vi "堆芯装卸料图程序.vi"() -> ()   [LabVIEW 2020]
doc: "图片控件可作为用户的绘图界面。本范例主要使用了画笔宽度和样式属性以及子集获取功能。子集获取是指从任意图像中截取一个矩形区域并绘制新图像的功能。"
uses:
  <vilib>/Utility/miscctls.llb/LVRowAndColumnTypeDef.ctl
  <vilib>/Analysis/baseanly.llb/Mean (DBL).vi
  GlobalVariable.vi
  <vilib>/Analysis/NI_AALBase.lvlib
panel:
  in  "操作显示":bool
  out "鼠标列":i32
  out "鼠标指示位置":i32(ring) items=["A"=0, "B"=1, "C"=2, "D"=3, "E"=4, "F"=5, "G"=6, "H"=7, "J"=8, "K"=9, "L"=10, "M"=11, "N"=12, " "=-2, " "=-1]
  in  "操作选项卡":enum32{"装卸料操作", "图操作"}(tab)
  in  "选取数据":bool
  out "波形图":dbl[][](graph)
  in  "当前堆内组件数":i32
  in  "SRC1&SRC2":string[][](array[string])
  in  "Select Pen Attributes":T1={"Width"=1, "Style"=enum."Solid"} caption="手动标记"
  out "Subset":picture caption="局部截图"
  in  "Select Operation":T2(ring) caption="选择操作"
  in  "Pen Color":u32(colorbox)=15671808 caption="标记颜色"
  out "Mouse Position.X":i32
  out "Mouse Position.Y":i32
  out "图层保存":bool
  in  "上一步装料":bool
  in  "下一步装料":bool
  out "PlanTable":string[][](table) caption="汇总表格"
  in  "初始化堆芯图":bool
  in  "保存图与SRC":bool
  out "Draw??":bool caption="绘制？？"
  out "Initial Coordinates":cluster{"Horizontal":i16, "Vertical":i16} caption="初始坐标"
  in  "退出程序":bool caption="停止"
  out "Picture":picture caption="堆芯图"
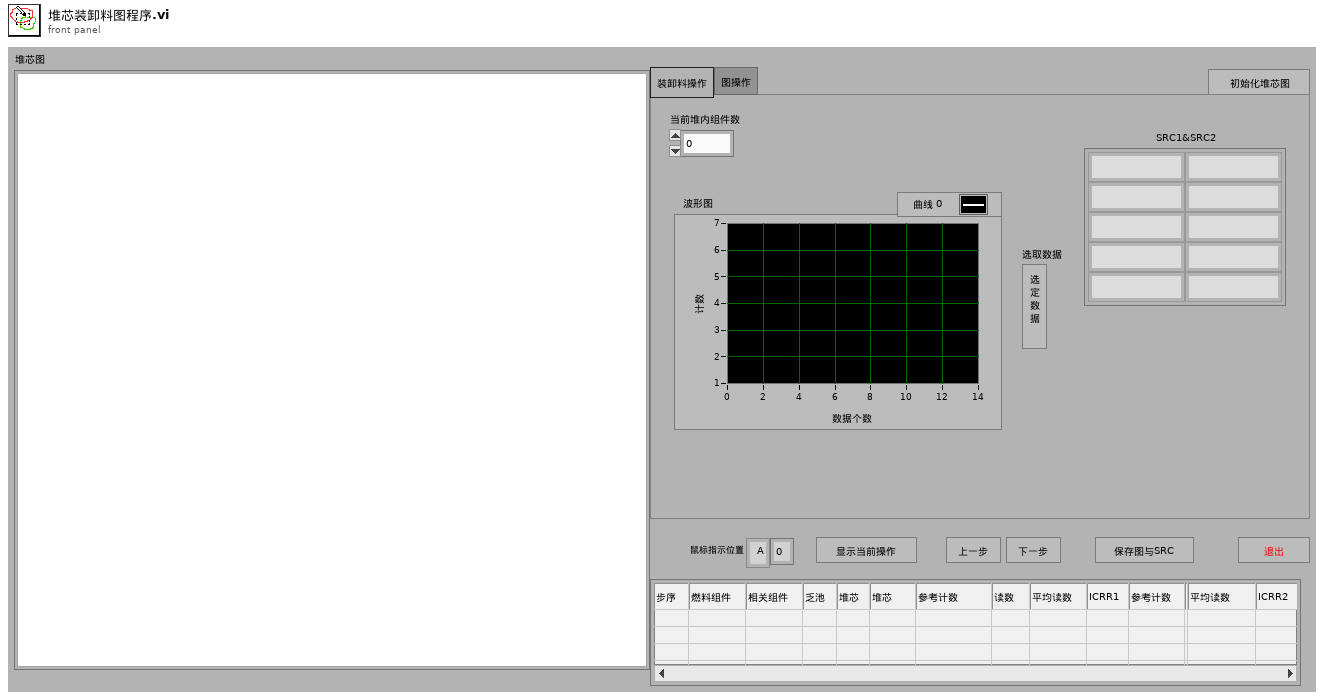
[diagram p1: front panel]
types:
  T1 = cluster{"Width":u16, "Style":enum32{"Solid", "Dash", "Dot", "DashDot", "DashDotDot"}}
  T2 = enum16{"Select Subset", "Draw Line", "Draw Point"}
  T3 = typedef "imagedata.ctl" = cluster{"image type":i32, "image depth":i32, "image":u8[], "mask":u8[], "colors":u32[], "Rectangle":cluster{"left":i16, "top":i16, "right":i16, "bottom":i16}}
  T4 = enum32{"Solid", "Dash", "Dot", "DashDot", "DashDotDot"}
  T5 = typedef "LVMouseTypeDef.ctl" = cluster{"Mouse Position":cluster{"X":i32, "Y":i32}, "Mouse Modifiers":cluster{"Button Down":bool, "Shift Mod":bool, "Menu Mod":bool, "Option Mod":bool}}
  T6 = typedef "LVRowAndColumnTypeDef.ctl" = cluster{"Row":i32, "Column":i32}
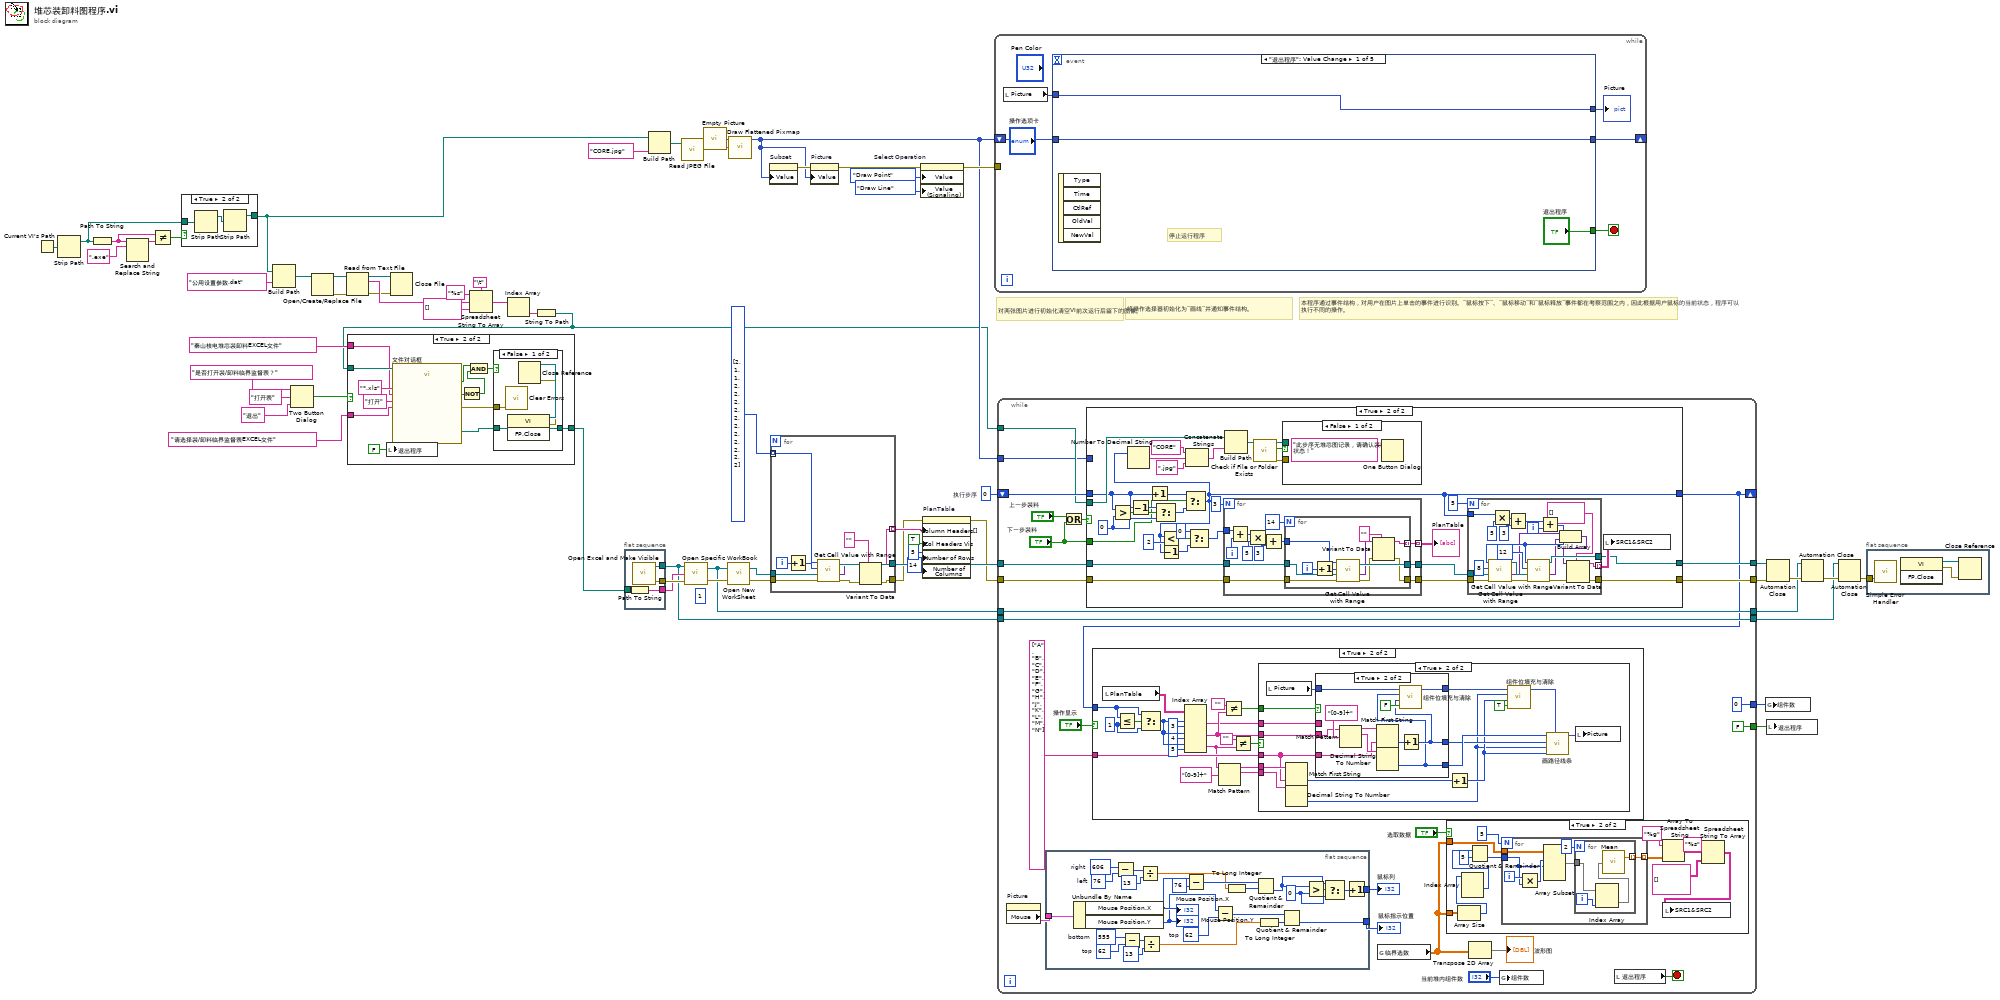
[diagram p0: block diagram]
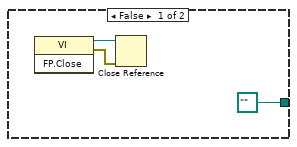
[diagram p2: hidden frame]
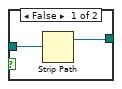
[diagram p4: hidden frame]
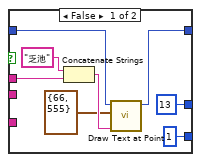
[diagram p8: hidden frame]
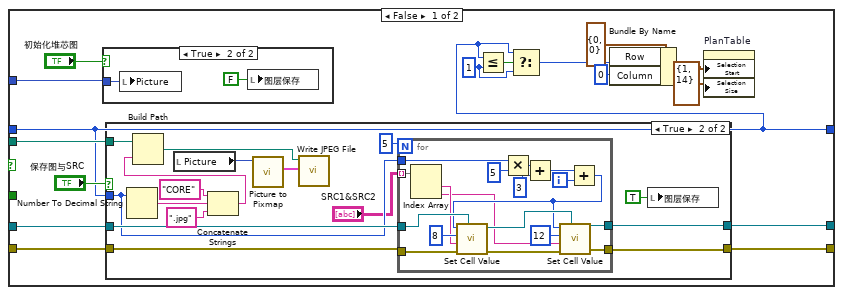
[diagram p9: hidden frame]
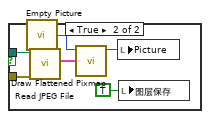
[diagram p12: hidden frame]
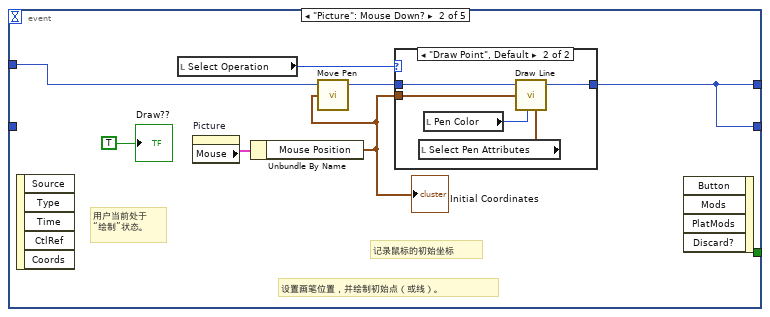
[diagram p13: hidden frame]
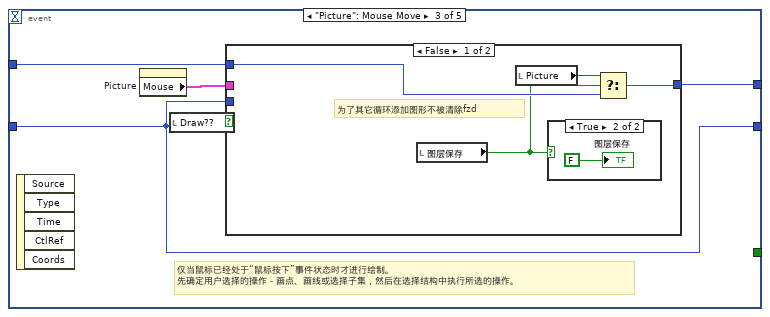
[diagram p15: hidden frame]
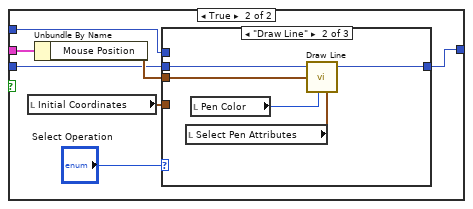
[diagram p17: hidden frame]
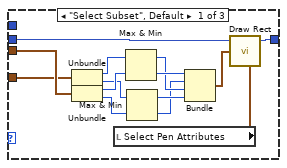
[diagram p18: hidden frame]
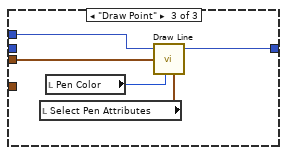
[diagram p19: hidden frame]
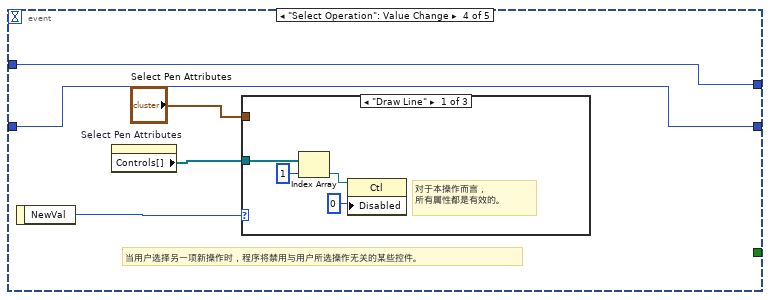
[diagram p20: hidden frame]
diagram:
  w32 = 0  # 执行步序
  (unwired) 1 ("Sheet")
  # "本程序通过事件结构，对用户在图片上单击的事件进行识别。“鼠标按下”、“鼠标移动”和“鼠标释放”事件都在考察范围之内，因此根据用户鼠标的当前状态，程序可以执行不同的操作。"
  # "将操作选择器初始化为“画线”并通知事件结构。"
  # "对两张图片进行初始化清空VI前次运行后留下的图像。"
  n1 = Current VI's Path() -> (path=w27:path)
  n2 = Strip Path(path=w27) -> (stripped path=w22:path)  [unwired: 1 out]
  n3 = Path To String(path=w22) -> (string=w24:string)
  n4 = Search and Replace String(input string=w24, search string=".exe" ("搜索字符串")) -> (result string=w25:string)  [unwired: 6 in, 3 out]
  n5 = Not Equal?(x=w24, y=w25) -> (x != y?=w23:bool)
  n6 = case shown="True" w23 {
    tunnel: w22 -> [w64 w67]
    tunnel: [w63 w65] -> w3
    frame False {
      n7 = Strip Path(path=w64) -> (stripped path=w63:path)  [unwired: 1 out]
    }
    frame True {
      n8 = Strip Path(path=w67) -> (stripped path=w66:path)  [unwired: 1 out]
      n9 = Strip Path(path=w66) -> (stripped path=w65:path)  [unwired: 1 out]
    }
  }
  n10 = Build Path(base path=w3, name or relative path="公用设置参数.dat") -> (appended path=w9:path)
  n11 = Two Button Dialog(message="是否打开装/卸料临界监督表？", 1:"退出" ("message"), 2:"打开表" ("message")) -> (T button?=w19:bool)
  n12 = Open/Create/Replace File(file path (use dialog)=w9) -> (refnum out=w12:refnum<file>, error out=w13:errorcluster)  [unwired: 5 in, 1 out]
  n13 = Read from Text File(file (use dialog)=w12, error in=w13) -> (refnum out=w11:refnum<file>, text=w17:string, error out=w10:errorcluster)  [unwired: 1 in, 2 out]
  n14 = Close File(refnum=w11, error in=w10) -> ()  [unwired: 2 out]
  n15 = Spreadsheet String To Array(delimiter (Tab)="\t", format string="%s", spreadsheet string=w17, array type (2D Dbl)=string[] [] ("添加的数组")) -> (array=w18:string[])
  n16 = Index Array(array=w18) -> (element=w7:string)  [unwired: 1 in]
  n17 = String To Path(string=w7) -> (path=w2:path)
  n18 = case shown="True" w19 {
    tunnel: w2 -> [_ w83]
    tunnel: "请选择装/卸料临界监督表EXCEL文件" ("prompt") -> [_ w79]
    tunnel: "秦山核电堆芯装卸料EXCEL文件" ("pattern label") -> [_ w78]
    tunnel: [path "" ("selected path") w76] -> w1
    frame False {
      n19 = invoke class="VI" method="FP.Close"() -> (reference out=w69:refnum<vi>, error out=w68:errorcluster)  [unwired: 3 in, 1 out]
      n20 = Close Reference(reference=w69, error in (no error)=w68) -> ()  [unwired: 1 out]
    }
    frame True {
      n21 = local write "退出程序"(FALSE ("退出程序")) -> ()
      n22 = call "文件对话框"("start path"=w83, "prompt"=w79, "button label"="打开", "pattern (all files)"="*.xls", "pattern label"=w78) -> ("selected path"=w77:path, "exists"=w74:bool, "cancelled"=w75:bool, "error out"=w71:errorcluster)  [unwired: 7 in]
      n23 = Not(x=w75) -> (.not. x?=w73:bool)
      n24 = And(x=w74, y=w73) -> (x .and. y?=w72:bool)
      n25 = case shown="False" w72 {
        tunnel: w77 -> [w87 w88]
        tunnel: [w87 w88] -> w76
        tunnel: w71 -> [w86 _]
        frame False {
          n26 = call <vilib>:"Clear Errors.vi"("error in (no error)"=w86) -> ()  [unwired: 5 in, 2 out]
          n27 = invoke class="VI" method="FP.Close"() -> (reference out=w85:refnum<vi>, error out=w84:errorcluster)  [unwired: 3 in, 1 out]
          n28 = Close Reference(reference=w85, error in (no error)=w84) -> ()  [unwired: 1 out]
        }
        frame True {
        }
      }
    }
  }
  n29 = flat-sequence {
    tunnel: [w92] -> w53
    tunnel: [w91] -> w52
    tunnel: [w90] -> w46
    tunnel: w1 -> [w89]
    frame #0 {
      n30 = Path To String(path=w89) -> (string=w91:string)
      n31 = call "Open Excel and Make Visible.vi"() -> ("error out"=w92:errorcluster, "Excel._Application"=w90:refnum<k7>)  [unwired: 2 in]
    }
  }
  n32 = Build Path(base path=w3, name or relative path="CORE.jpg" ("名称或相对路径")) -> (appended path=w57:path)
  n33 = call <vilib>:"Read JPEG File.vi"("path to JPEG file"=w57) -> ("image data"=w55:T3)  [unwired: 8 in, 2 out]
  n34 = call "Open Specific WorkBook.vi"("error in (no error)"=w53, "Filename of Workbook"=w52, "Excel._Application"=w46) -> ("error out"=w43:errorcluster, "Excel._Workbook"=w42:refnum<k7>)
  n35 = call "Empty Picture"() -> ("empty picture"=w54:picture)
  n36 = call "Open New WorkSheet.vi"("error in (no error)"=w43, "Excel._Workbook"=w42) -> ("error out"=w40:errorcluster, "Excel._Worksheet"=w38:refnum<k7>)  [unwired: 1 in]
  n37 = call <vilib>:"Draw Flattened Pixmap.vi"("image data"=w55, "picture"=w54) -> ("new picture"=w41:picture)  [unwired: 7 in]
  n38 = property on="Subset" class="Pict"("Value"=w41) -> (error out=w58:errorcluster)  [unwired: 2 in, 1 out]
  n39 = for {
    tunnel: w40 -> [w103]
    tunnel: [w95] -> w34
    tunnel: [w102] -> w39
    tunnel: w38 -> [w101]
    tunnel: i32[] [2, 1, 1, 2, 2, 2, 2, 2, 2, 2, 2, 2, 2, 2] -> [w98] mode=indexing
    tunnel: [w93] -> w35 mode=indexing
    i -> [w100]
    n40 = Increment(x=w100) -> (x+1=w99:i32)
    n41 = call "Get Cell Value with Range.vi"("error in (no error)"=w103, "Excel._Worksheet"=w101, "Col"=w99, "Row"=w98) -> ("error out"=w96:errorcluster, "Data Out"=w97:variant, "Excel._Worksheet"=w102:refnum<k7>)  [unwired: 1 out]
    n42 = Variant To Data(error in=w96, type="" ("Workbook Name"), Variant=w97) -> (data=w93:string, error out=w95:errorcluster)
  }
  n43 = property on="Picture" class="Pict"(error in=w58, "Value"=w41) -> (error out=w59:errorcluster)  [unwired: 1 in, 1 out]
  n44 = property on="Select Operation" class="Enum (strict)"(error in=w59, "Value"=T2."Draw Point" ("Select Your Operation"), "Value (Signaling)"=T2."Draw Line" ("Select Your Operation")) -> (error out=w62:errorcluster)  [unwired: 1 in, 1 out]
  n45 = property on="PlanTable" class="Tbl (strict)"(error in=w34, "Column Headers[]"=w35, "Col Headers Vis"=TRUE ("显示项:显示列首"), "Number of Rows"=u32 5 ("行数"), "Number of Columns"=u32 14 ("列数")) -> (error out=w33:errorcluster)  [unwired: 1 in, 1 out]
  n46 = while {
    shift-right: [w105] -> _
    shift-left: w41 -> [w104]
    tunnel: w62 -> [_]
    stop <- w108 stop-if-true
    n47 = local read "Picture"() -> (w107:picture)
    n48 = event shown="[0] \"退出程序\": Value Change" {
      selector: _ -> [_ _ _ _ _]
      dyn-events: _ -> [_ _ _ _ _]
      timeout: _ -> [_ _ _ _ _]
      tunnel: ["退出程序" _ _ _ _] -> w108
      tunnel: [w110 w114 w127 w169 w189] -> w106
      tunnel: w107 -> [w110 w116 w126 w169 w191]
      tunnel: [w109 w114 w125 w166 w189] -> w105
      tunnel: w104 -> [w109 _ w125 w166 w190]
      event "退出程序": Value Change {
        # "停止运行程序"
        n49 = event-data() -> ()  [unwired: 1 in, 5 out]
      }
      event "Picture": Mouse Down? {
        # "设置画笔位置，并绘制初始点（或线）。"
        # "记录鼠标的初始坐标"
        # "用户当前处于\n“绘制”状态。"
        n50 = event-data() -> ()  [unwired: 1 in, 5 out]
        n51 = local read "Select Operation"() -> (w112:T2)
        n52 = property on="Picture" class="Pict"() -> ("Mouse"=w118:T5)  [unwired: 2 in, 2 out]
        n53 = Unbundle By Name(w118) -> ("Mouse Position"=w113:cluster{"X":i32, "Y":i32})
        "Initial Coordinates" <- w113
        n54 = call <vilib>:"Move Pen.vi"("new position"=w113, "picture"=w116) -> ("new picture"=w115:picture)  [unwired: 3 in]
        n55 = case shown="\"Draw Point\", Default" w112 {
          tunnel: w115 -> [w119 w124]
          tunnel: [w119 w123] -> w114
          tunnel: w113 -> [_ w122]
          frame "Select Subset" {
          }
          frame "Draw Point", Default {
            n56 = local read "Select Pen Attributes"() -> (w121:T1)
            n57 = local read "Pen Color"() -> (w120:u32)
            n58 = call <vilib>:"Draw Line.vi"("picture"=w124, "end point"=w122, "color(black)"=w120, "pen"=w121) -> ("new picture"=w123:picture)  [unwired: 5 in]
          }
        }
        n59 = event-data() -> ()  [unwired: 5 in, 1 out]
        "Draw??" <- TRUE ("Draw??")
      }
      event "Picture": Mouse Move {
        # "仅当鼠标已经处于“鼠标按下”事件状态时才进行绘制。\n先确定用户选择的操作－画点、画线或选择子集，然后在选择结构中执行所选的操作。"
        n60 = event-data() -> ()  [unwired: 1 in, 5 out]
        n61 = property on="Picture" class="Pict"() -> ("Mouse"=w128:T5)  [unwired: 2 in, 2 out]
        n62 = local read "Draw??"() -> (w129:bool)
        n63 = case shown="False" w129 {
          tunnel: w126 -> [w132 w140]
          tunnel: w128 -> [_ w139]
          tunnel: [w133 w136] -> w127
          tunnel: w125 -> [_ w135]
          frame False {
            # "为了其它循环添加图形不被清除fzd"
            n64 = local read "图层保存"() -> (w130:bool)
            n65 = local read "Picture"() -> (w131:picture)
            n66 = case shown="True" w130 {
              frame False {
              }
              frame True {
                "图层保存" <- FALSE ("图层保存")
              }
            }
            n67 = Select(t=w131, s=w130, f=w132) -> (s? t:f=w133:picture)
          }
          frame True {
            n68 = local read "Initial Coordinates"() -> (w138:cluster{"Horizontal":i16, "Vertical":i16})
            n69 = Unbundle By Name(w139) -> ("Mouse Position"=w137:cluster{"X":i32, "Y":i32})
            n70 = case shown="\"Draw Line\"" "Select Operation" {
              tunnel: w140 -> [_ _ w162]
              tunnel: w138 -> [w154 _ _]
              tunnel: w137 -> [w155 w159 w163]
              tunnel: [w152 w160 w165] -> w136
              tunnel: w135 -> [w151 w157 _]
              frame "Select Subset", Default {
                n71 = Unbundle(w154) -> ("Horizontal"=w149:i16, "Vertical"=w145:i16)
                n72 = Unbundle(w155) -> ("X"=w148:i32, "Y"=w144:i32)
                n73 = local read "Select Pen Attributes"() -> (w150:T1)
                n74 = Max & Min(x=w149, y=w148) -> (max(x,y)=w146:i32, min(x,y)=w147:i32)
                n75 = Max & Min(x=w145, y=w144) -> (max(x,y)=w143:i32, min(x,y)=w142:i32)
                n76 = Bundle(w147, w142, w146, w143) -> (w153:cluster{i32, i32, i32, i32})  [unwired: 1 in]
                n77 = call <vilib>:"Draw Rect.vi"("picture"=w151, "rect"=w153, "pen"=w150) -> ("new picture"=w152:picture)  [unwired: 6 in]
              }
              frame "Draw Line" {
                n78 = local read "Select Pen Attributes"() -> (w158:T1)
                n79 = local read "Pen Color"() -> (w156:u32)
                n80 = call <vilib>:"Draw Line.vi"("picture"=w157, "end point"=w159, "color(black)"=w156, "pen"=w158) -> ("new picture"=w160:picture)  [unwired: 5 in]
              }
              frame "Draw Point" {
                n81 = local read "Select Pen Attributes"() -> (w164:T1)
                n82 = local read "Pen Color"() -> (w161:u32)
                n83 = call <vilib>:"Draw Line.vi"("picture"=w162, "end point"=w163, "color(black)"=w161, "pen"=w164) -> ("new picture"=w165:picture)  [unwired: 5 in]
              }
            }
          }
        }
      }
      event "Select Operation": Value Change {
        # "当用户选择另一项新操作时，程序将禁用与用户所选操作无关的某些控件。"
        n84 = event-data() -> ("NewVal"=w170:T2)  [unwired: 1 in]
        n85 = property on="Select Pen Attributes" class="Clust (strict)"() -> ("Controls[]"=w168:refnum<vi>[])  [unwired: 2 in, 2 out]
        n86 = case shown="\"Draw Line\"" w170 {
          tunnel: w168 -> [w174 w181 w188]
          tunnel: "Select Pen Attributes" -> [_ w176 w183]
          frame "Draw Line" {
            # "对于本操作而言，\n所有属性都是有效的。"
            n87 = Index Array(array=w174, index=1) -> (element=w172:refnum<vi>)
            n88 = property class="Ctl"(reference=w172, "Disabled"=u8 0) -> ()  [unwired: 1 in, 2 out]
          }
          frame "Draw Point" {
            # "样式属性与本操作无关。\n因此可以禁用该控件\n并将其值锁定于Solid。"
            n89 = Index Array(array=w181, index=1) -> (element=w179:refnum<vi>)
            n90 = Bundle By Name(cluster=w176, "Style"=T4."Solid") -> (w175:T1)
            n91 = property class="Ctl"(reference=w179, "Disabled"=u8 2) -> ()  [unwired: 1 in, 2 out]
            n92 = property on="Select Pen Attributes" class="Clust (strict)"("Value"=w175) -> ()  [unwired: 2 in, 2 out]
          }
          frame "Select Subset" {
            # "用户选择子集时，程序将选框样式锁定于Dash。"
            n93 = Index Array(array=w188, index=1) -> (element=w186:refnum<vi>)
            n94 = Bundle By Name(cluster=w183, "Style"=T4."Dash") -> (w182:T1)
            n95 = property class="Ctl"(reference=w186, "Disabled"=u8 2) -> ()  [unwired: 1 in, 2 out]
            n96 = property on="Select Pen Attributes" class="Clust (strict)"("Value"=w182) -> ()  [unwired: 2 in, 2 out]
          }
        }
      }
      event "Picture": Mouse Up {
        # "用户绘制完毕后，程序完成该项操作。只需要完成该项操作，\n“选择子集”操作就全部完成了。"
        # "绘制完成"
        n97 = event-data() -> ()  [unwired: 1 in, 1 out]
        n98 = local read "Select Operation"() -> (w193:T2)
        n99 = local write "Draw??"(FALSE ("Draw??")) -> ()
        n100 = case shown="\"Draw Point\"" w193 {
          tunnel: w191 -> [_ w210 w211]
          tunnel: [w194 w210 w211] -> w189
          tunnel: w190 -> [w194 _ _]
          frame "Select Subset", Default {
            # "获取选框的坐标，然后从主图片中抽取子集，并在子集显示控件中\n将该子集绘制为一张新图片。"
            n101 = local read "Initial Coordinates"() -> (w207:cluster{"Horizontal":i16, "Vertical":i16})
            n102 = property on="Picture" class="Pict"() -> ("Mouse"=w208:T5)  [unwired: 2 in, 2 out]
            n103 = Unbundle By Name(w208) -> ("Mouse Position.X"=w197:i32, "Mouse Position.Y"=w195:i32)
            n104 = Unbundle By Name(w207) -> ("Horizontal"=w198:i16, "Vertical"=w196:i16)
            n105 = Max & Min(x=w198, y=w197) -> (max(x,y)=w202:i32, min(x,y)=w201:i32)
            n106 = Max & Min(x=w196, y=w195) -> (max(x,y)=w200:i32, min(x,y)=w199:i32)
            n107 = call <vilib>:"Picture to Pixmap.vi"("picture"=w194) -> ("image data"=w209:T3)  [unwired: 9 in, 1 out]
            n108 = Bundle(w201, w199, w202, w200) -> (w206:cluster{i32, i32, i32, i32})  [unwired: 1 in]
            n109 = call <vilib>:"Get Image Subset.vi"("subset rect"=w206, "image data"=w209) -> ("image subset"=w205:T3)  [unwired: 4 in, 1 out]
            n110 = call "Empty Picture"() -> ("empty picture"=w203:picture)
            n111 = call <vilib>:"Draw Flattened Pixmap.vi"("image data"=w205, "picture"=w203) -> ("new picture"=→"Subset":picture)  [unwired: 7 in]
          }
          frame "Draw Line" {
          }
          frame "Draw Point" {
          }
        }
      }
    }
    "Picture" <- w106
  }
  n112 = while {
    tunnel: [w236] -> w48
    tunnel: [w235] -> w45
    tunnel: [w234] -> w47
    tunnel: w39 -> [w233]
    tunnel: w46 -> [w234]
    tunnel: [w231] -> w44
    tunnel: w33 -> [w232]
    tunnel: w42 -> [w231]
    tunnel: w41 -> [w224]
    shift-right: [w214] -> _
    shift-left: w32 -> [w226]
    tunnel: w2 -> [w225]
    tunnel: [0 ("组件数")] -> w31
    tunnel: [FALSE ("退出程序")] -> w30
    stop <- w220 stop-if-true
    n113 = property on="Picture" class="Pict"() -> ("Mouse"=w230:T5)  [unwired: 2 in, 2 out]
    n114 = flat-sequence {
      tunnel: w230 -> [w285]
      tunnel: [w266] -> w218
      tunnel: [w261] -> w217
      frame #0 {
        w263 = 0 ("y")
        w271 = i16 555  # bottom
        w268 = i16 62  # top
        w272 = i16 62  # top
        w275 = i16 606  # right
        w274 = i16 76  # left
        n115 = Unbundle By Name(w285) -> ("Mouse Position.X"=w284:i32, "Mouse Position.Y"=w283:i32)
        "Mouse Position.X" <- w284
        "Mouse Position.Y" <- w283
        n116 = Subtract(x=w275, y=w274) -> (x-y=w276:i16)
        n117 = Subtract(x=w271, y=w268) -> (x-y=w269:i16)
        n118 = Divide(x=w276, y=i16 13) -> (x/y=w273:dbl)
        n119 = Divide(x=w269, y=i16 13) -> (x/y=w267:dbl)
        n120 = Subtract(x=w284, y=76) -> (x-y=w282:i32)
        n121 = Subtract(x=w283, y=w272) -> (x-y=w281:i32)
        n122 = To Long Integer(number=w273) -> (32bit integer=w279:i32)
        n123 = Quotient & Remainder(x=w282, y=w279) -> (floor(x/y)=w264:i32)  [unwired: 1 out]
        n124 = To Long Integer(number=w267) -> (32bit integer=w280:i32)
        n125 = Quotient & Remainder(x=w281, y=w280) -> (floor(x/y)=w266:i32)  [unwired: 1 out]
        n126 = Greater?(x=w264, y=w263) -> (0:w265:bool)
        n127 = Select(t=w264, s=w265, f=w263) -> (s? t:f=w262:i32)
        n128 = Increment(x=w262) -> (x+1=w261:i32)
      }
    }
    n129 = Or(x="上一步装料", y="下一步装料") -> (x .or. y?=w228:bool)
    n130 = case shown="True" w228 {
      tunnel: [w351 w415] -> w236
      tunnel: [w350 w406] -> w235
      tunnel: w233 -> [w353 w425]
      tunnel: w232 -> [w352 w424]
      tunnel: w226 -> [w341 w396]
      tunnel: [w341 w394] -> w214
      tunnel: "下一步装料" -> [_ w408]
      tunnel: w225 -> [w354 w401]
      tunnel: w224 -> [w348 _]
      frame False {
        w343 = 1 ("y")
        n131 = case shown="True" "初始化堆芯图" {
          tunnel: w348 -> [_ w357]
          frame False {
          }
          frame True {
            n132 = local write "Picture"(w357) -> ()
            n133 = local write "图层保存"(FALSE ("图层保存")) -> ()
          }
        }
        n134 = case shown="True" "保存图与SRC" {
          tunnel: w341 -> [_ w362]
          tunnel: w354 -> [_ w373]
          tunnel: w353 -> [w358 w367]
          tunnel: w352 -> [w359 w365]
          tunnel: [w359 w366] -> w351
          tunnel: [w358 w363] -> w350
          frame False {
          }
          frame True {
            n135 = Number To Decimal String(number=w362) -> (decimal integer string=w371:string)  [unwired: 1 in]
            n136 = local read "Picture"() -> (w374:picture)
            n137 = Concatenate Strings("CORE" ("字符串"), w371, ".jpg" ("字符串")) -> (w369:string)
            n138 = Build Path(base path=w373, name or relative path=w369) -> (appended path=w368:path)
            n139 = call <vilib>:"Picture to Pixmap.vi"("picture"=w374) -> ("image data"=w375:T3)  [unwired: 9 in, 1 out]
            n140 = call <vilib>:"Write JPEG File.vi"("image data"=w375, "path to JPEG file"=w368) -> ()  [unwired: 8 in, 2 out]
            n141 = for {
              N: 5 -> [_]
              tunnel: w365 -> [w393]
              tunnel: w367 -> [w392]
              tunnel: [w381] -> w366
              tunnel: [w389] -> w363
              tunnel: w362 -> [w380]
              tunnel: "SRC1&SRC2" -> [w379] mode=indexing
              i -> [w382]
              n142 = Index Array(array=w379) -> (element #1=w377:string, element #2=w376:string)  [unwired: 2 in]
              n143 = Multiply(x=w380, y=5) -> (x*y=w385:i32)
              n144 = Add(x=w385, y=3) -> (x+y=w383:i32)
              n145 = Add(x=w383, y=w382) -> (x+y=w378:i32)
              n146 = call "Set Cell Value.vi"("Excel._Worksheet"=w392, "error in (no error)"=w393, 6:w377, "Col"=8, "Row"=w378) -> ("error out"=w391:errorcluster, "Excel._Worksheet"=w390:refnum<k7>)  [unwired: 1 in, 1 out]
              n147 = call "Set Cell Value.vi"("Excel._Worksheet"=w390, "error in (no error)"=w391, 6:w376, "Col"=12, "Row"=w378) -> ("error out"=w381:errorcluster, "Excel._Worksheet"=w389:refnum<k7>)  [unwired: 1 in, 1 out]
            }
            n148 = local write "图层保存"(TRUE ("图层保存")) -> ()
          }
        }
        n149 = Less Or Equal?(x=w341, y=w343) -> (x <= y?=w342:bool)
        n150 = Select(t=w341, s=w342, f=w343) -> (s? t:f=w340:i32)
        n151 = Bundle By Name(cluster=T6 {"Row"=0, "Column"=0} ("选择区域起始"), "Row"=w340, "Column"=0) -> (w345:T6)
        n152 = property on="PlanTable" class="Tbl (strict)"("Selection Start"=w345, "Selection Size"=T6 {"Row"=1, "Column"=14} ("选择区域大小")) -> ()  [unwired: 2 in, 2 out]
      }
      frame True {
        w420 = 0 ("y")
        n153 = Greater?(x=w396, y=w420) -> (0:w422:bool)
        n154 = Decrement(x=w396) -> (x-1=w421:i32)
        n155 = Increment(x=w396) -> (x+1=w423:i32)
        n156 = Select(t=w421, s=w422, f=w420) -> (s? t:f=w419:i32)
        n157 = Select(t=w423, s=w408, f=w419) -> (s? t:f=w394:i32)
        n158 = Number To Decimal String(number=w394) -> (decimal integer string=w403:string)  [unwired: 1 in]
        n159 = Less?(x=w394, y=2) -> (x < y?=w412:bool)
        n160 = Decrement(x=w394) -> (x-1=w409:i32)
        n161 = Concatenate Strings("CORE" ("字符串"), w403, ".jpg" ("字符串")) -> (w405:string)
        n162 = Select(t=0 ("y"), s=w412, f=w409) -> (s? t:f=w410:i32)
        n163 = for {
          N: 3 -> [_]
          tunnel: [w466] -> w417
          tunnel: [w465] -> w416
          tunnel: w425 -> [w464]
          tunnel: w424 -> [w463]
          tunnel: [w461] -> w395 mode=indexing
          tunnel: w410 -> [w454]
          i -> [w460]
          n164 = Add(x=w454, y=w460) -> (x+y=w455:i32)
          n165 = Multiply(x=w455, y=5) -> (x*y=w458:i32)
          n166 = Add(x=w458, y=3) -> (x+y=w456:i32)
          n167 = for {
            N: 14 -> [_]
            tunnel: [w468] -> w466
            tunnel: [w477] -> w465
            tunnel: w464 -> [w476]
            tunnel: w463 -> [w475]
            tunnel: w456 -> [w472]
            tunnel: [w467] -> w461 mode=indexing
            i -> [w473]
            n168 = Increment(x=w473) -> (x+1=w474:i32)
            n169 = call "Get Cell Value with Range.vi"("error in (no error)"=w475, "Excel._Worksheet"=w476, "Col"=w474, "Row"=w472) -> ("error out"=w469:errorcluster, "Data Out"=w470:variant, "Excel._Worksheet"=w477:refnum<k7>)  [unwired: 1 out]
            n170 = Variant To Data(error in=w469, type="" ("Workbook Name"), Variant=w470) -> (data=w467:string, error out=w468:errorcluster)
          }
        }
        "PlanTable" <- w395
        n171 = Build Path(base path=w401, name or relative path=w405) -> (appended path=w400:path)
        n172 = call <vilib>:"Check if File or Folder Exists.vi"("path"=w400) -> ("error out"=w398:errorcluster, "file or folder exists?"=w397:bool, "dup path"=w399:path)  [unwired: 8 in]
        n173 = case shown="False" w397 {
          tunnel: w399 -> [_ w430]
          tunnel: w398 -> [_ w429]
          frame False {
            n174 = One Button Dialog(message="此步序无堆芯图记录，请确认装料状态！" ("消息")) -> ()  [unwired: 1 in, 1 out]
          }
          frame True {
            n175 = call "Empty Picture"() -> ("empty picture"=w431:picture)
            n176 = call <vilib>:"Read JPEG File.vi"("error in (no error)"=w429, "path to JPEG file"=w430) -> ("image data"=w432:T3)  [unwired: 7 in, 2 out]
            n177 = call <vilib>:"Draw Flattened Pixmap.vi"("image data"=w432, "picture"=w431) -> ("new picture"=w428:picture)  [unwired: 7 in]
            n178 = local write "Picture"(w428) -> ()
            n179 = local write "图层保存"(TRUE ("图层保存")) -> ()
          }
        }
        n180 = for {
          N: 5 -> [_]
          tunnel: w417 -> [w453]
          tunnel: w416 -> [w452]
          tunnel: [w448] -> w415
          tunnel: [w447] -> w406
          tunnel: w394 -> [w441]
          tunnel: [w433] -> w407 mode=indexing
          i -> [w439]
          n181 = Multiply(x=w441, y=5) -> (x*y=w443:i32)
          n182 = Add(x=w443, y=3) -> (x+y=w440:i32)
          n183 = Add(x=w440, y=w439) -> (x+y=w438:i32)
          n184 = call "Get Cell Value with Range.vi"("error in (no error)"=w453, "Excel._Worksheet"=w452, "Col"=8, "Row"=w438) -> ("error out"=w451:errorcluster, "Data Out"=w437:variant, "Excel._Worksheet"=w450:refnum<k7>)  [unwired: 1 out]
          n185 = call "Get Cell Value with Range.vi"("error in (no error)"=w451, "Excel._Worksheet"=w450, "Col"=12, "Row"=w438) -> ("error out"=w449:errorcluster, "Data Out"=w436:variant, "Excel._Worksheet"=w447:refnum<k7>)  [unwired: 1 out]
          n186 = Build Array(w437, w436) -> (w435:variant[])
          n187 = Variant To Data(error in=w449, type=string[] [], Variant=w435) -> (data=w433:string[], error out=w448:errorcluster)
        }
        n188 = local write "SRC1&SRC2"(w407) -> ()
      }
    }
    n189 = case shown="True" "操作显示" {
      tunnel: string[] ["A", "B", "C", "D", "E", "F", "G", "H", "J", "K", "L", "M", "N"] -> [_ w291]
      tunnel: w214 -> [_ w289]
      frame False {
      }
      frame True {
        w293 = 1 ("y")
        n190 = local read "PlanTable"() -> (w290:string[][])
        n191 = Less Or Equal?(x=w289, y=w293) -> (x <= y?=w292:bool)
        n192 = Select(t=w289, s=w292, f=w293) -> (s? t:f=w294:i32)
        n193 = Index Array(array=w290, index (row) #1=w294, index (col) #1=3 ("禁用的索引 (列)"), index (row) #2=w294, index (col) #2=4 ("禁用的索引 (列)"), index (row) #3=w294, index (col) #3=5 ("禁用的索引 (列)")) -> (element #1=w301:string, element #2=w303:string, element #3=w287:string)
        n194 = Match Pattern(string=w287, regular expression="[0-9]+" ("正则表达式")) -> (before substring=w299:string, match substring=w300:string)  [unwired: 1 in, 2 out]
        n195 = Not Equal?(x="", y=w303) -> (x != y?=w304:bool)
        n196 = Not Equal?(x="", y=w287) -> (x != y?=w286:bool)
        n197 = case shown="True" w286 {
          tunnel: w304 -> [_ w317]
          tunnel: w303 -> [_ w316]
          tunnel: w301 -> [_ w315]
          tunnel: w300 -> [_ w313]
          tunnel: w299 -> [_ w312]
          tunnel: w291 -> [_ w311]
          frame False {
          }
          frame True {
            n198 = local read "Picture"() -> (w310:picture)
            n199 = Match First String ("匹配字符串")(2:w311, 3:w312) -> (0:w320:i32)  [unwired: 1 out]
            n200 = Decimal String To Number(string=w313) -> (number=w305:i32)  [unwired: 2 in, 1 out]
            n201 = case shown="True" w317 {
              tunnel: w311 -> [_ w336]
              tunnel: w316 -> [_ w335]
              tunnel: w315 -> [w326 _]
              tunnel: [13 ("index") w330] -> w318
              tunnel: [1 w329] -> w319
              tunnel: w310 -> [w322 w333]
              tunnel: [w321 w331] -> w309
              frame False {
                n202 = Concatenate Strings("乏池" ("字符串"), w326) -> (w324:string)
                n203 = call <vilib>:"Draw Text at Point.vi"("text"=w324, "origin"=cluster{"x":i16, "y":i16} {"x"=66, "y"=555}, "picture"=w322) -> ("new picture"=w321:picture)  [unwired: 7 in, 1 out]
              }
              frame True {
                n204 = Match Pattern(string=w335, regular expression="[0-9]+" ("正则表达式")) -> (before substring=w338:string, match substring=w337:string)  [unwired: 1 in, 2 out]
                n205 = Match First String(2:w336, 3:w338) -> (0:w334:i32)  [unwired: 1 out]
                n206 = Decimal String To Number(string=w337) -> (number=w329:i32)  [unwired: 2 in, 1 out]
                n207 = Increment(x=w334) -> (x+1=w330:i32)
                n208 = call "组件位填充与清除.vi"("添/清"=FALSE, "行字母"=w330, "列数字"=w329, "PictureIN"=w333) -> ("PictureOUT"=w331:picture)  [unwired: 7 in]
              }
            }
            n209 = Increment(x=w320) -> (x+1=w306:i32)
            n210 = call "组件位填充与清除.vi"("添/清"=TRUE, "行字母"=w306, "列数字"=w305, "PictureIN"=w309) -> ("PictureOUT"=w308:picture)  [unwired: 7 in]
            n211 = call "画路径线条.vi"("图片输入"=w308, "结束行"=w306, "结束列"=w305, "开始行"=w318, "开始列"=w319) -> ("图片输出"=w314:picture)  [unwired: 6 in]
            n212 = local write "Picture"(w314) -> ()
          }
        }
      }
    }
    n213 = global read "GlobalVariable.vi" "临界选数"() -> (w212:dbl[][])
    n214 = case shown="True" "选取数据" {
      tunnel: w212 -> [_ w249]
      tunnel: w212 -> [_ w245]
      frame False {
      }
      frame True {
        n215 = Array Size(array=w249) -> (size(s)=w248:i32[])
        n216 = Index Array(array=w248) -> (element #1=w247:i32)  [unwired: 2 in, 1 out]
        n217 = Quotient & Remainder(x=w247, y=5) -> (floor(x/y)=w243:i32)  [unwired: 1 out]
        n218 = for {
          N: 5 -> [_]
          tunnel: w245 -> [w256]
          tunnel: w243 -> [w251]
          tunnel: [w252] -> w242 mode=indexing
          i -> [w255]
          n219 = Multiply(x=w255, y=w251) -> (x*y=w254:i32)
          n220 = Array Subset(array=w256, index (row)=w254, length (row)=w251) -> (w253:dbl[][])  [unwired: 2 in]
          n221 = for {
            N: 2 -> [_]
            tunnel: w253 -> [w259]
            tunnel: [w260] -> w252 mode=indexing
            i -> [w257]
            n222 = Index Array(array=w259, index (col)=w257) -> (element=w258:dbl[])  [unwired: 1 in]
            n223 = call-poly <vilib>:"Mean.vi"("X"=w258) -> ("mean"=w260:dbl)  [unwired: 1 out]
          }
        }
        n224 = Array To Spreadsheet String(array=w242, 3:"%g" ("格式字符串")) -> (spreadsheet string=w240:string)  [unwired: 1 in]
        n225 = Spreadsheet String To Array(format string="%s" ("格式字符串"), spreadsheet string=w240, array type (2D Dbl)=string[][] []) -> (array=w237:string[][])  [unwired: 1 in]
        n226 = local write "SRC1&SRC2"(w237) -> ()
      }
    }
    n227 = Transpose 2D Array(2D array=w212) -> (transposed array=→"波形图":dbl[][])
    n228 = global write "GlobalVariable.vi" "组件数"("当前堆内组件数") -> ()
    n229 = local read "退出程序"() -> (w220:bool)
    "鼠标列" <- w217
    "鼠标指示位置" <- w218
  }
  n230 = global write "GlobalVariable.vi" "组件数"(w31) -> ()
  n231 = local write "退出程序"(w30) -> ()
  n232 = Automation Close(3:w48, 5:w45) -> (0:w51:errorcluster)
  n233 = Automation Close(3:w51, 5:w44) -> (0:w50:errorcluster)
  n234 = Automation Close(3:w50, 5:w47) -> (0:w49:errorcluster)
  n235 = flat-sequence {
    tunnel: w49 -> [w480]
    frame #0 {
      n236 = call <vilib>:"Simple Error Handler.vi"("error in (no error)"=w480) -> ()  [unwired: 4 in, 5 out]
      n237 = invoke class="VI" method="FP.Close"() -> (reference out=w479:refnum<vi>, error out=w478:errorcluster)  [unwired: 3 in, 1 out]
      n238 = Close Reference(reference=w479, error in (no error)=w478) -> ()  [unwired: 1 out]
    }
  }
